vi "generate_unique_filename.vi"(10 "Filename (no extension)":string, 11 "Data Folder":path) -> (2 "Filename":path)   [LabVIEW 2016]
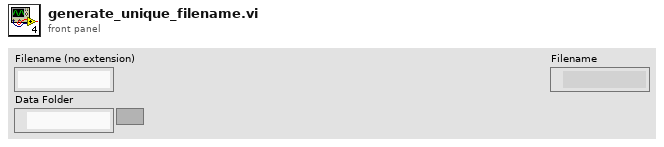
[diagram p1: front panel]
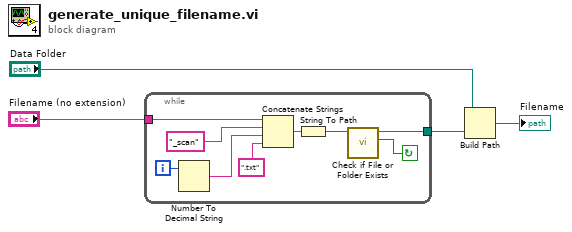
[diagram p0: block diagram]
diagram:
  n1 = while {
    tunnel: "Filename (no extension)" -> [w13]
    tunnel: [w5] -> w3
    i -> [w11]
    stop <- w6 continue-if-true
    n2 = Number To Decimal String(number=w11) -> (decimal integer string=w10:string)  [unwired: 1 in]
    n3 = Concatenate Strings(w13, "_scan", w10, ".txt") -> (w7:string)
    n4 = String To Path(string=w7) -> (path=w8:path)
    n5 = call <vilib>:"Check if File or Folder Exists.vi"("path"=w8) -> ("file or folder exists?"=w6:bool, "dup path"=w5:path)  [unwired: 8 in, 1 out]
  }
  n6 = Build Path(base path="Data Folder", name or relative path=w3) -> (appended path=→"Filename":path)
